vi "Globals_Settings_XLP80.vi"() -> ()   [LabVIEW 2021]
uses:
  XLP80_Datalog/XLP80_Datalog_TypeDefEnumLogselect.ctl
  <userlib>/PCAN Basic/Controls/Channel.ctl
  XLP80_General_Libs/Kirschenhofer_Libs/KH_DAQ 17.04/KH_DAQ_TypeDefs_Cluster AI.ctl
  XLP80_General_Libs/Kirschenhofer_Libs/KH_DAQ 17.04/KH_DAQ_TypeDefs_Messbereich.ctl
  XLP80_General_Libs/Kirschenhofer_Libs/KH EthernetIPConfig 17.14/KH EthernetIPConfig TypeDefs ModuleTyp.ctl
  XLP80_General_Libs/Kirschenhofer_Libs/KH_DAQ 17.04/KH_DAQ_TypeDefs_Bereich.ctl
  XLP80_General_Libs/Kirschenhofer_Libs/KH_DAQ 17.04/KH_DAQ_TypeDefs_Cluster AO.ctl
  XLP80_General_Libs/Kirschenhofer_Libs/KH_DAQ 17.04/Turck/KH_DAQ_TURCK_TypeDefs_Cluster DI.ctl
  XLP80_General_Libs/Kirschenhofer_Libs/KH_DAQ 17.04/Turck/KH_DAQ_TURCK_TypeDefs_Cluster DO.ctl
  <userlib>/PCAN Basic/PCANBasic.lvlib
panel:
  in  "Settings":T1(tab)=enum."Datalog"
  in  "EthernetIP ConfigFile":path=path "C:/Template/Results"
  in  "LogFile Path":path=path "C:/Template/Results"
  in  "Result Path":path=path "C:/Template/Results"
  in  "Settings Path":path=path "C:/Template/Settings"
  in  "MaxFileSize":i32
  in  "Logselect":T2[](array[typedef])
  in  "CVM Parameter":T3={"CVM Graph"={"CVM Warning"=0.0, "CVM Alarm"=0.0, "CVM GraphMin"=0.0, "CVM GraphMax"=0.0}, "Cells"=10, "StartChannel"="", "CVM Simulate"=TRUE, "CVMSimulation"={"CVMin"=0.0, "CVPeakNoise"=0.0}} {"CVMSimulation"."CVPeakNoise" min=0 max=1 scale=0.0..0.1; "CVMSimulation"."CVMin" min=0 max=1 scale=0.0..1.0}
  in  "ReadData":T4={"SheetName"="Header", "OffsetData"=2, "StartCell"="A3", "EndColumn"="D"}
  in  "ReadMetaData":T5={"SheetName"="Metadata", "NoOfRows"=6, "StartCell"="A1"}
  in  "Alarm Table Real":T6 {"Ena" format="%04b"; "Limits_III" format="%.2e"; "Limits II" format="%.2e"; "Limits I" format="%.2e"; "Index" max=63}
  in  "Alarm Table Bool":T7 {"Ena" format="%04b"; "Index" max=63}
  in  "EIP_AI":T8 {"Offset" format="%.4f"; "Phys Max" format="%.4f"; "Phys Min" format="%.4f"}
  in  "EIP_AO":T12 {"Offset" format="%.4f"; "Phys Max" format="%.4f"; "Phys Min" format="%.4f"}
  in  "EIP_DI":T13 {"Nr" max=63; "Chan" max=63}
  in  "EIP_DO":T14 {"Nr" max=63; "Chan" max=63}
  in  "CAN DBC":path
  in  "Peak Channel":T15=enum."PCAN_PCIBUS1"
  in  "Settings_CANWrite_Testmode_B":T16={"Signal Name"=["LV_en_p_cldn_amblimit_temp", "LV_en_p_cldn_amblimitoff_temp", "LV_en_p_cldn_cp_spd", "LV_en_p_cldn_rf_spd", "LV_en_p_cldn_rf_time", "LV_en_p_cldn_soclimit", "LV_en_p_cldn_time2off", "LV_en_p_cvm_diff_maxmin_lim", "LV_en_p_cvm_frequency", "LV_en_p_cvm_low_lim2", "LV_en_p_cvm_temperature", "LV_en_p_cvm_up_lim1", "LV_en_p_cvm_up_lim2", "LV_en_p_fcsd_etc_initrng_spd", "LV_en_p_fcsd_h2end_press", "LV_en_p_fcsd_hrbstp_spd", "LV_en_p_fcsu_bpv_opncls_time", "LV_en_p_fcsu_dcdc_currrampgrad", "LV_en_p_fcsu_dcdc_maxwrmup_curr", "LV_en_p_fcsu_dcdc_optime", "LV_en_p_fcsu_dcdc_preoptime", "LV_en_p_fcsu_etc_initspd", "LV_en_p_fcsu_ghu_strtpress1", "LV_en_p_fcsu_ghu_strtpress2", "LV_en_p_fcsu_h2_initpress", "LV_en_p_fcsu_h2_strtpress", "LV_en_p_fcsu_hrb_strtspd", "LV_en_p_fcsu_initmincellvolt", "LV_en_p_fcsu_mincellvolt_time", "LV_en_p_fcsu_pvrmp_incrclstime", "LV_en_p_fcsu_pvrmp_opntime", "LV_en_p_fcsu_pvrmp_strtclstime", "LV_en_p_fcsu_stk_deltamedlow_v", "LV_en_p_fcsu_stk_lowcellvolt", "LV_en_p_fcsu_stk_normopset_temp", "LV_en_p_hmi_bat_soc_limit_low", "LV_en_p_hmi_bat_soc_limit_ok", "LV_en_p_hmi_h2_leak_amb_ppm", "LV_en_p_hmi_h2_leak_exh_ppm", "LV_en_p_hmi_h2_leak_exh_s", "LV_en_p_hmi_h2tanklvl_displ", "LV_en_p_hmi_h2tanklvl_presslim", "LV_en_p_hmi_h2tanklvl_scale0", "LV_en_p_hmi_h2tanklvl_scale1", "LV_en_p_hrbo_a_valve_async_fact", "LV_en_p_hrbo_a_valve_i_fact", "LV_en_p_hrbo_a_valve_ot_fact", "LV_en_p_p_minucell_range1_time", "LV_en_p_p_minucell_range1_volt", "LV_en_p_p_minucell_range2_time", "LV_en_p_p_minucell_range2_volt", "LV_en_p_pc_uirangecell_time", "LV_en_p_pc_uirangecell_volt", "LV_en_p_power_out_fc_high", "LV_en_p_power_out_fc_low", "LV_en_p_rfc_hghvent_fanspd", "LV_en_p_rfc_nrmopbaseval_fanspd", "LV_en_p_rfc_srtstpvent_fanspd", "LV_en_p_soc_limit_fc_high", "LV_en_p_soc_limit_fc_low", "LV_en_p_soc_limit_fc_off", "LV_en_p_spdn_batlimit_curr", "LV_en_p_spdn_batlimit_time", "LV_en_p_tc_clpmpspd_idx0", "LV_en_p_tc_clpmpspd_idx1", "LV_en_p_tc_clpmpspd_idx2", "LV_en_P_TC_GHU_maxlowpress", "LV_en_P_TC_GHU_maxmidpress", "LV_en_P_TC_OTV_maxtankpress", "LV_en_p_wtlc_soc_lvl_perc", "LV_en_p_wtlc_soc_time2off_sec", "LV_P_CLDN_AMBlimit_Temp", "LV_P_CLDN_AMBlimitOff_Temp", "LV_P_CLDN_CP_Spd", "LV_P_CLDN_RF_Spd", "LV_P_CLDN_RF_Time", "LV_P_CLDN_SOClimit", "LV_P_CLDN_time2off", "LV_P_CVM_Diff_MaxMin_Lim", "LV_P_CVM_Frequency", "LV_P_CVM_Low_Lim2", "LV_P_CVM_Temperature", "LV_P_CVM_Up_Lim1", "LV_P_CVM_Up_Lim2", "LV_P_FCSD_ETC_InitRng_Spd", "LV_P_FCSD_H2end_Press", "LV_P_FCSD_HRBstp_Spd", "LV_P_FCSU_BPV_OpnCls_Time", "LV_P_FCSU_DCDC_CurrRampGrad", "LV_P_FCSU_DCDC_MaxWrmUp_Curr", "LV_P_FCSU_DCDC_OpTime", "LV_P_FCSU_DCDC_PreOpTime", "LV_P_FCSU_ETC_InitSpd", "LV_P_FCSU_GHU_StrtPress1", "LV_P_FCSU_GHU_StrtPress2", "LV_P_FCSU_H2_InitPress", "LV_P_FCSU_H2_Press_I_Ctrl", "LV_P_FCSU_H2_Press_P_Ctrl", "LV_P_FCSU_H2_StrtPress", "LV_P_FCSU_HRB_StrtSpd", "LV_P_FCSU_InitMinCellVolt", "LV_P_FCSU_MinCellVolt_Time", "LV_P_FCSU_PVrmp_IncrClsTime", "LV_P_FCSU_PVrmp_IniOpnTime", "LV_P_FCSU_PVrmp_StrtClsTime", "LV_P_FCSU_STK_DeltaMedLow_V", "LV_P_FCSU_STK_LowCellVolt", "LV_P_FCSU_STK_NormOpSet_Temp", "LV_P_HMI_BAT_SOC_Limit_low", "LV_P_HMI_BAT_SOC_Limit_ok", "LV_P_HMI_H2_leak_amb_ppm", "LV_P_HMI_H2_leak_exh_ppm", "LV_P_HMI_H2_leak_exh_s", "LV_P_HMI_H2TankLvl_Displ", "LV_P_HMI_H2TankLvl_PressLim", "LV_P_HMI_H2TankLvl_Scale0", "LV_P_HMI_H2TankLvl_Scale1", "LV_P_HRBo_a_Valve_Async_fact", "LV_P_HRBo_a_Valve_I_fact", "LV_P_HRBo_a_Valve_OT_fact", "LV_P_PC_MinUCell_range1_Time", "LV_P_PC_MinUCell_range1_Volt", "LV_P_PC_MinUCell_range2_Time", "LV_P_PC_MinUCell_range2_Volt", "LV_P_PC_UIrangeCell_Time", "LV_P_PC_UIrangeCell_Volt", "LV_P_Power_Out_FC_High", "LV_P_Power_Out_FC_Low", "LV_P_RFC_HghVent_FanSpd", "LV_P_RFC_NrmOpBaseVal_FanSpd", "LV_P_RFC_SrtStpVent_FanSpd", "LV_P_SOC_Limit_FC_High", "LV_P_SOC_Limit_FC_Low", "LV_P_SOC_Limit_FC_Off", "LV_P_SPDN_BATlimit_Curr", "LV_P_SPDN_BATlimit_Time", "LV_P_TC_ClPmpSpd_Amp0", "LV_P_TC_ClPmpSpd_Amp1", "LV_P_TC_ClPmpSpd_Amp2", "LV_P_TC_ClPmpSpd_perc0", "LV_P_TC_ClPmpSpd_perc1", "LV_P_TC_ClPmpSpd_perc2", "LV_P_TC_GHU_MaxLowPress", "LV_P_TC_GHU_MaxMidPress", "LV_P_TC_OTV_MaxTankPress", "LV_P_TC_StkIntT_I_Crtl_FanSpd", "LV_P_TC_StkIntT_P_Crtl_FanSpd", "LV_P_WTLC_SOC_Lvl", "LV_P_WTLC_SOC_time2off", "LV_Testmode_Select", "S80_BP_s_Taster_Start_Status", "S80_BP_s_Taster_Stop_Status"], "Description"=["", "", "", "", "", "", "", "", "", "", "", "", "", "", "", "", "", "", "", "", "", "", "", "", "", "", "", "", "", "", "", "", "", "", "", "", "", "", "", "", "", "", "", "", "", "", "", "", "", "", "", "", "", "", "", "", "", "", "", "", "", "", "", "", "", "", "", "", "", "", "", "", "", "", "", "", "", "", "", "", "", "", "", "", "", "", "", "", "", "", "", "", "", "", "", "", "", "", "", "", "", "", "", "", "", "", "", "", "", "", "", "", "", "", "", "", "", "", "", "", "", "", "", "", "", "", "", "", "", "", "", "", "", "", "", "", "", "", "", "", "", "", "", "", "", "", "", "", "", "", "", ""], "Unit"=["", "", "", "", "", "", "", "", "", "", "", "", "", "", "", "", "", "", "", "", "", "", "", "", "", "", "", "", "", "", "", "", "", "", "", "", "", "", "", "", "", "", "", "", "", "", "", "", "", "", "", "", "", "", "", "", "", "", "", "", "", "", "", "", "", "", "", "", "", "", "", "°C", "°C", "%", "%", "s", "%", "s", "V", "Hz", "V", "°C", "V", "V", "rpm", "kPa", "rpm", "s", "A/s", "A", "s", "s", "rpm", "kPa", "kPa", "kPa", "", "", "kPa", "rpm", "V", "s", "s", "s", "s", "V", "V", "°C", "%", "%", "ppm", "ppm", "s", "%", "kPa", "kPa", "kPa", "", "", "", "s", "V", "s", "V", "s", "V", "A", "A", "%", "%", "%", "%", "%", "%", "A", "s", "A", "A", "A", "%", "%", "%", "kPa", "kPa", "kPa", "", "", "%", "s", "", "", ""], "Default"=[0.0, 0.0, 0.0, 0.0, 0.0, 0.0, 0.0, 0.0, 0.0, 0.0, 0.0, 0.0, 0.0, 0.0, 0.0, 0.0, 0.0, 0.0, 0.0, 0.0, 0.0, 0.0, 0.0, 0.0, 0.0, 0.0, 0.0, 0.0, 0.0, 0.0, 0.0, 0.0, 0.0, 0.0, 0.0, 0.0, 0.0, 0.0, 0.0, 0.0, 0.0, 0.0, 0.0, 0.0, 0.0, 0.0, 0.0, 0.0, 0.0, 0.0, 0.0, 0.0, 0.0, 0.0, 0.0, 0.0, 0.0, 0.0, 0.0, 0.0, 0.0, 0.0, 0.0, 0.0, 0.0, 0.0, 0.0, 0.0, 0.0, 0.0, 0.0, 0.0, 0.0, 0.0, 0.0, 0.0, 0.0, 0.0, 0.0, 0.0, 0.0, 0.0, 0.0, 0.0, 0.0, 0.0, 0.0, 0.0, 0.0, 0.0, 0.0, 0.0, 0.0, 0.0, 0.0, 0.0, 0.0, 0.0, 0.0, 0.0, 0.0, 0.0, 0.0, 0.0, 0.0, 0.0, 0.0, 0.0, 0.0, 0.0, 0.0, 0.0, 0.0, 0.0, 0.0, 0.0, 0.0, 0.0, 0.0, 0.0, 0.0, 0.0, 0.0, 0.0, 0.0, 0.0, 0.0, 0.0, 0.0, 0.0, 0.0, 0.0, 0.0, 0.0, 0.0, 0.0, 0.0, 0.0, 0.0, 0.0, 0.0, 0.0, 0.0, 0.0, 0.0, 0.0, 0.0, 0.0, 0.0, 0.0, 0.0, 0.0], "Min"=[0.0, 0.0, 0.0, 0.0, 0.0, 0.0, 0.0, 0.0, 0.0, 0.0, 0.0, 0.0, 0.0, 0.0, 0.0, 0.0, 0.0, 0.0, 0.0, 0.0, 0.0, 0.0, 0.0, 0.0, 0.0, 0.0, 0.0, 0.0, 0.0, 0.0, 0.0, 0.0, 0.0, 0.0, 0.0, 0.0, 0.0, 0.0, 0.0, 0.0, 0.0, 0.0, 0.0, 0.0, 0.0, 0.0, 0.0, 0.0, 0.0, 0.0, 0.0, 0.0, 0.0, 0.0, 0.0, 0.0, 0.0, 0.0, 0.0, 0.0, 0.0, 0.0, 0.0, 0.0, 0.0, 0.0, 0.0, 0.0, 0.0, 0.0, 0.0, 0.0, 0.0, 0.0, 0.0, 0.0, 0.0, 0.0, 0.0, 0.0, 0.0, 0.0, 0.0, 0.0, 0.0, 0.0, 0.0, 0.0, 0.0, 0.0, 0.0, 0.0, 0.0, 0.0, 0.0, 0.0, 0.0, 0.0, 0.0, 0.0, 0.0, 0.0, 0.0, 0.0, 0.0, 0.0, 0.0, 0.0, 0.0, 0.0, 0.0, 0.0, 0.0, 0.0, 0.0, 0.0, 0.0, 0.0, 0.0, 0.0, 0.0, 0.0, 0.0, 0.0, 0.0, 0.0, 0.0, 0.0, 0.0, 0.0, 0.0, 0.0, 0.0, 0.0, 0.0, 0.0, 0.0, 0.0, 0.0, 0.0, 0.0, 0.0, 0.0, 0.0, 0.0, 0.0, 0.0, 0.0, 0.0, 0.0, 0.0, 0.0], "Max"=[100.0, 100.0, 100.0, 100.0, 100.0, 100.0, 100.0, 100.0, 100.0, 100.0, 100.0, 100.0, 100.0, 100.0, 100.0, 100.0, 100.0, 100.0, 100.0, 100.0, 100.0, 100.0, 100.0, 100.0, 100.0, 100.0, 100.0, 100.0, 100.0, 100.0, 100.0, 100.0, 100.0, 100.0, 100.0, 100.0, 100.0, 100.0, 100.0, 100.0, 100.0, 100.0, 100.0, 100.0, 100.0, 100.0, 100.0, 100.0, 100.0, 100.0, 100.0, 100.0, 100.0, 100.0, 100.0, 100.0, 100.0, 100.0, 100.0, 100.0, 100.0, 100.0, 100.0, 100.0, 100.0, 100.0, 100.0, 100.0, 100.0, 100.0, 100.0, 100.0, 100.0, 100.0, 100.0, 100.0, 100.0, 100.0, 100.0, 100.0, 100.0, 100.0, 100.0, 100.0, 100.0, 100.0, 100.0, 100.0, 100.0, 100.0, 100.0, 100.0, 100.0, 100.0, 100.0, 100.0, 100.0, 100.0, 100.0, 100.0, 100.0, 100.0, 100.0, 100.0, 100.0, 100.0, 100.0, 100.0, 100.0, 100.0, 100.0, 100.0, 100.0, 100.0, 100.0, 100.0, 100.0, 100.0, 100.0, 100.0, 100.0, 100.0, 100.0, 100.0, 100.0, 100.0, 100.0, 100.0, 100.0, 100.0, 100.0, 100.0, 100.0, 100.0, 100.0, 100.0, 100.0, 100.0, 100.0, 100.0, 100.0, 100.0, 100.0, 100.0, 100.0, 100.0, 100.0, 100.0, 100.0, 100.0, 100.0, 100.0], "Preconditions"=[FALSE, FALSE, FALSE, FALSE, FALSE, FALSE, FALSE, FALSE, FALSE, FALSE, FALSE, FALSE, FALSE, FALSE, FALSE, FALSE, FALSE, FALSE, FALSE, FALSE, FALSE, FALSE, FALSE, FALSE, FALSE], "HV & Software"=[FALSE, FALSE, FALSE, FALSE, FALSE, FALSE, FALSE, FALSE, FALSE, FALSE, FALSE, FALSE, FALSE, FALSE, FALSE, FALSE, FALSE, FALSE, FALSE, FALSE, FALSE, FALSE, FALSE, FALSE, FALSE], "Basis Funktion"=[FALSE, FALSE, FALSE, FALSE, FALSE, FALSE, FALSE, FALSE, FALSE, FALSE, FALSE, FALSE, FALSE, FALSE, FALSE, FALSE, FALSE, FALSE, FALSE, FALSE, FALSE, FALSE, FALSE, FALSE, FALSE], "Power Management"=[FALSE, FALSE, FALSE, FALSE, FALSE, FALSE, FALSE, FALSE, FALSE, FALSE, FALSE, FALSE, FALSE, FALSE, FALSE, FALSE, FALSE, FALSE, FALSE, FALSE, FALSE, FALSE, FALSE, FALSE, FALSE], "OperationMode"=[FALSE, FALSE, FALSE, FALSE, FALSE, FALSE, FALSE, FALSE, FALSE, FALSE, FALSE, FALSE, FALSE, FALSE, FALSE, FALSE, FALSE, FALSE, FALSE, FALSE, FALSE, FALSE, FALSE, FALSE, FALSE], "Shutdown"=[FALSE, FALSE, FALSE, FALSE, FALSE, FALSE, FALSE, FALSE, FALSE, FALSE, FALSE, FALSE, FALSE, FALSE, FALSE, FALSE, FALSE, FALSE, FALSE, FALSE, FALSE, FALSE, FALSE, FALSE, FALSE], "Alarm"=[FALSE, FALSE, FALSE, FALSE, FALSE, FALSE, FALSE, FALSE, FALSE, FALSE, FALSE, FALSE, FALSE, FALSE, FALSE, FALSE, FALSE, FALSE, FALSE, FALSE, FALSE, FALSE, FALSE, FALSE, FALSE], "LogEnable"=[FALSE, FALSE, FALSE, FALSE, FALSE, FALSE, FALSE, FALSE, FALSE, FALSE, FALSE, FALSE, FALSE, FALSE, FALSE, FALSE, FALSE, FALSE, FALSE, FALSE, FALSE, FALSE, FALSE, FALSE, FALSE]} {"Max" format="%.2f"; "Min" format="%.2f"; "Default" format="%.2f"}
  in  "Settings_CANRead_Testmode_B":T17 {"Max" format="%.2f"; "Min" format="%.2f"}
  in  "Settings_CANWrite_Testmode_A":T18={"Signal Name"=["LV_A_03_ETC_a_opCmd1_Error_Ack", "LV_A_03_ETC_a_opCmd1_Start_Stop", "LV_A_03_ETC_a_Speed_Set", "LV_A_11_HBV_a_Valve_Enable", "LV_A_11_HBV_a_Valve_Set", "LV_A_12_SIV_a_Valve_Enable", "LV_A_12_SIV_a_Valve_Set", "LV_A_13_SOV_a_Valve_Enable", "LV_A_13_SOV_a_Valve_Set", "LV_C_01_RF_a_FanSpeed", "LV_C_02_CP_a_RPM", "LV_E_74_ISO_a_Rq_D_IMC_STEST_SCR", "LV_E_75_HVP_a_Relais_Set", "LV_E_76_HVM_a_Relais_Set", "LV_H_31_OTV_a_Valve_Set", "LV_H_38_HSV_a_Valve_Set", "LV_H_42_HRB_a_FCCU_Spd_Rq", "LV_H_42_HRB_a_KNF_Speed_Rq", "LV_H_43_HDV_a_Dosing_Valve_Set", "LV_H_46_HRBo_a_Drain_Valve_Set", "LV_H_52_DV_a_Drain_Valve_Stack", "LV_H_53_PV_a_Purge_Valve_Stack", "LV_Testmode_Select", "S80_BP_s_Taster_Start_Status", "S80_BP_s_Taster_Stop_Status"], "Description"=["", "", "", "", "", "", "", "", "", "", "", "", "", "", "", "", "", "", "", "", "", "", "", "", ""], "Unit"=["", "", "rpm", "", "%", "", "%", "", "%", "%", "%", "", "", "", "", "", "rpm", "%", "%", "", "", "", "", "", ""], "Default"=[0.0, 0.0, 0.0, 0.0, 0.0, 0.0, 0.0, 0.0, 0.0, 0.0, 0.0, 0.0, 0.0, 0.0, 0.0, 0.0, 0.0, 0.0, 0.0, 0.0, 0.0, 0.0, 0.0, 0.0, 0.0], "Min"=[0.0, 0.0, 0.0, 0.0, 0.0, 0.0, 0.0, 0.0, 0.0, 0.0, 0.0, 0.0, 0.0, 0.0, 0.0, 0.0, 0.0, 0.0, 0.0, 0.0, 0.0, 0.0, 0.0, 0.0, 0.0], "Max"=[100.0, 100.0, 100.0, 100.0, 100.0, 100.0, 100.0, 100.0, 100.0, 100.0, 100.0, 100.0, 100.0, 100.0, 100.0, 100.0, 100.0, 100.0, 100.0, 100.0, 100.0, 100.0, 100.0, 100.0, 100.0], "TestmodeA"=[FALSE, FALSE, FALSE, FALSE, FALSE, FALSE, FALSE, FALSE, FALSE, FALSE, FALSE, FALSE, FALSE, FALSE, FALSE, FALSE, FALSE, FALSE, FALSE, FALSE, FALSE, FALSE, FALSE, FALSE, FALSE], "LogEnable"=[FALSE, FALSE, FALSE, FALSE, FALSE, FALSE, FALSE, FALSE, FALSE, FALSE, FALSE, FALSE, FALSE, FALSE, FALSE, FALSE, FALSE, FALSE, FALSE, FALSE, FALSE, FALSE, FALSE, FALSE, FALSE]} {"Max" format="%.2f"; "Min" format="%.2f"; "Default" format="%.2f"}
  in  "Settings_CANRead_Testmode_A":T19={"Signal Name"=["A03_ETC_a_CAN_Set_Baudrate", "A03_ETC_a_CAN_Set_Broadcast", "A03_ETC_a_CAN_Set_ID_Offset", "A03_ETC_a_CAN_Set_Termination", "A03_ETC_a_CAN_Set_Timeout", "A03_ETC_a_CAN_Set_Timeout_Dur", "A03_ETC_a_Diag_Rq_Select", "A03_ETC_a_Info_Rq_Select", "A03_ETC_a_opCmd1_Error_Ack", "A03_ETC_a_opCmd1_Start_Stop", "A03_ETC_a_opCmd2", "A03_ETC_a_Param_Rq_Select", "A03_ETC_a_Speed_Set", "A03_ETC_s_ArticleNumber", "A03_ETC_s_ArticleRevision", "A03_ETC_s_BootloaderVersion", "A03_ETC_s_Converter_Temperature", "A03_ETC_s_Diag_Select", "A03_ETC_s_Error_Code_1", "A03_ETC_s_Error_Code_2", "A03_ETC_s_FirmwareVersion", "A03_ETC_s_GasBearingCondition", "A03_ETC_s_HV_In_Voltage", "A03_ETC_s_Info_Select", "A03_ETC_s_Information_Code", "A03_ETC_s_LV_In_Voltage", "A03_ETC_s_Output_Power", "A03_ETC_s_Phase_Current", "A03_ETC_s_Phase_Current_Ref", "A03_ETC_s_Phase_Voltage", "A03_ETC_s_PT100_Temperature", "A03_ETC_s_Serial_Part_1", "A03_ETC_s_Serial_Part_2", "A03_ETC_s_Serial_Part_3", "A03_ETC_s_Speed_Actual", "A03_ETC_s_Speed_Reference", "A03_ETC_s_Status1", "A03_ETC_s_Status2", "A03_ETC_s_THC_Temperature", "A03_ETC_s_Warning_Code", "A11_HBV_a_Mode_Set", "A11_HBV_a_Valve_Set", "A11_HBV_s_Mode_Act", "A11_HBV_s_Valve_Act", "A12_SIV_a_Mode_Set", "A12_SIV_a_Valve_Set", "A12_SIV_s_Mode_Act", "A12_SIV_s_Valve_Act", "A13_SOV_a_Mode_Set", "A13_SOV_a_Valve_Set", "A13_SOV_s_Mode_Act", "A13_SOV_s_Valve_Act", "A14_HFM_s_AirMassFlow", "A14_HFM_s_Error_MassFlow", "A14_HFM_s_Error_Pressure", "A14_HFM_s_ErrorCode", "A14_HFM_s_Humidity", "A14_HFM_s_HumidTemperature", "A14_HFM_s_Pressure", "A14_HFM_s_Temperature", "A15_SI_s_Inlet_Pressure", "A16_SI_s_Inlet_Temperature", "A17_SO_s_Outlet_Pressure", "A17_SO_s_Outlet_Temperature", "A22_HSI_s_Humidity", "A23_HSO_s_Humidity", "A56_SO_s_Temperature", "C01_RF_a_FanSpeed", "C01_RF_s_Status", "C02_CP_a_RPM", "C04_DI_s_Temperature", "C06_ET_s_CoolLevelStatus", "C07_BAT_s_BatError_DataValid", "C07_BAT_s_BatError_Intern", "C07_BAT_s_BatError_Temperature", "C07_BAT_s_BatError_Voltage", "C07_BAT_s_Battery_Voltage", "C07_BAT_s_Board_Temperature", "C07_BAT_s_CECUError_Communicat", "C07_BAT_s_CECUError_Current", "C07_BAT_s_CECUError_Intern", "C07_BAT_s_CECUError_Reserved", "C07_BAT_s_CECUError_Service", "C07_BAT_s_CECUError_Supply", "C07_BAT_s_CECUError_Temperature", "C07_BAT_s_CECUError_Voltage", "C07_BAT_s_External_Chrg_Voltage", "C07_BAT_s_External_Load_Voltage", "C07_BAT_s_Max_Cell_Temperature", "C07_BAT_s_Max_Cell_Voltage", "C07_BAT_s_Min_Cell_Temperature", "C07_BAT_s_Min_Cell_Voltage", "C07_BAT_s_PreWarning_Current_H", "C07_BAT_s_PreWarning_SOC_Low", "C07_BAT_s_PreWarning_Temperature", "C07_BAT_s_PreWarning_Voltage_HL", "C07_BAT_s_State", "C07_BAT_s_System_Current", "C08_AMB_s_Humidity_Rel", "C08_AMB_s_Humidity_Spec", "C08_AMB_s_Pressure", "C08_AMB_s_Temperature", "C54_SI_s_Temperature", "C_07_BAT_s_SoC", "C_07_BAT_s_SoH", "E71_DC4880_a_Current_In_Set", "E71_DC4880_a_Current_Out_Set", "E71_DC4880_a_Mode_Control_On", "E71_DC4880_a_Mode_Precharge_On", "E71_DC4880_a_NMT_Function", "E71_DC4880_a_NMT_Node_ID", "E71_DC4880_a_Voltage_In_Set", "E71_DC4880_a_Voltage_Out_Set", "E71_DC4880_s_Current_In_Actual", "E71_DC4880_s_Current_Out_Actual", "E71_DC4880_s_NMT_State", "E71_DC4880_s_State_Control_OK", "E71_DC4880_s_State_Control_On", "E71_DC4880_s_State_Precharge_On", "E71_DC4880_s_Temperature_1_Act", "E71_DC4880_s_Temperature_2_Act", "E71_DC4880_s_Voltage_In_Actual", "E71_DC4880_s_Voltage_Out_Actual", "E72_DC8024_s_Voltage", "E73_DC8012_s_Voltage", "E74_ISO_a_CMD_Rq", "E74_ISO_a_Rq_D_IMC_MANUFACT_IDX", "E74_ISO_a_Rq_D_IMC_MEAN_FACTOR", "E74_ISO_a_Rq_D_IMC_R_ISOERR_THR", "E74_ISO_a_Rq_D_IMC_R_ISOWRN_THR", "E74_ISO_a_Rq_D_IMC_SELFTEST_SCR", "E74_ISO_a_Rq_D_IMC_VERSION_IDX", "E74_ISO_a_Rq_D_VIFC_HV_REL_CHG", "E74_ISO_a_Rq_D_VIFC_HV_RELAIS", "E74_ISO_a_Rq_D_VIFC_LOCK_MODE", "E74_ISO_a_Rq_D_VIFC_LOCK_PWD", "E74_ISO_a_Rq_D_VIFC_MEAS_MODE", "E74_ISO_a_Rq_D_VIFC_RELAIS_STAT", "E74_ISO_a_Rq_D_VIFC_VERSION_IDX", "E74_ISO_s_CMD_Resp", "E74_ISO_s_D_IMC_HV_1", "E74_ISO_s_D_IMC_HV_2", "E74_ISO_s_D_IMC_MANUFACT_DATA", "E74_ISO_s_D_IMC_MANUFACT_INDEX", "E74_ISO_s_D_IMC_MEAN_FACTOR", "E74_ISO_s_D_IMC_R_ISO", "E74_ISO_s_D_IMC_R_ISO_BIAS", "E74_ISO_s_D_IMC_R_ISO_CNT", "E74_ISO_s_D_IMC_R_ISO_ERR_THR1", "E74_ISO_s_D_IMC_R_ISO_ERR_THR2", "E74_ISO_s_D_IMC_R_ISO_WRN_THR1", "E74_ISO_s_D_IMC_R_ISO_WRN_THR2", "E74_ISO_s_D_IMC_SELFTEST_SCR", "E74_ISO_s_D_IMC_STATUS", "E74_ISO_s_D_IMC_STATUS_EXT", "E74_ISO_s_D_IMC_TEST_CNT", "E74_ISO_s_D_IMC_VERSION_Haupt", "E74_ISO_s_D_IMC_VERSION_INDEX", "E74_ISO_s_D_IMC_VERSION_Neben", "E74_ISO_s_D_IMD_ERROR_CODE", "E74_ISO_s_D_IMD_FAILED_CMD", "E74_ISO_s_D_VIFC_HV_RELAIS", "E74_ISO_s_D_VIFC_HV_RELAIS_ACT", "E74_ISO_s_D_VIFC_HV_RELAIS_CHG", "E74_ISO_s_D_VIFC_HV_RELAIS_STAT", "E74_ISO_s_D_VIFC_IMC_ALIVE", "E74_ISO_s_D_VIFC_LOCK_MODE", "E74_ISO_s_D_VIFC_MEASURE_MODE", "E74_ISO_s_D_VIFC_STATUS", "E74_ISO_s_D_VIFC_VERSION_Haupt", "E74_ISO_s_D_VIFC_VERSION_INDEX", "E74_ISO_s_D_VIFC_VERSION_Neben", "E74_ISO_s_IMC_R_ISO", "E74_ISO_s_IMC_STATUS_ErrChassis", "E74_ISO_s_IMC_STATUS_Isofehler", "E74_ISO_s_IMC_STATUS_Isowarnung", "E74_ISO_s_IMC_STATUS_Kalib", "E74_ISO_s_IMC_STATUS_Selbsttest", "E74_ISO_s_IMC_STATUS_Syststoer", "E74_ISO_s_Rq_D_IMC_MEAN_FACTOR", "E74_ISO_s_VIFC_STATUS_IMC_Alive", "E74_ISO_s_VIFC_STATUS_IMC_St_OA", "E74_ISO_s_VIFC_STATUS_IMC_St_PC", "E74_ISO_s_VIFC_STATUS_IsoAlt", "E74_ISO_s_VIFC_STATUS_Isomess", "E74_ISO_s_VIFC_STATUS_Stoer_IMC", "E74_ISO_s_VIFC_STATUS_VIFC_Cmd", "E75_HVP_a_Relais_Set", "E76_HVM_a_Relais_Set", "E95_DC2405_s_Voltage", "H31_OTV_a_Valve_Set", "H31_OTV_s_Pressure", "H31_OTV_s_Temperature", "H36_GHU_s_Pressure_1", "H37_GHU_s_Temperature_1", "H38_HSV_a_Valve_Set", "H40_GHU_s_Pressure_2", "H41_GHU_s_Temperature_2", "H42_HRB_a_FCCU_CRC", "H42_HRB_a_FCCU_Heating_Rq", "H42_HRB_a_FCCU_Spd_Rq", "H42_HRB_a_FCCU_SQC", "H42_HRB_s_ARB_Batt_Vltg_Err", "H42_HRB_s_ARB_Batt_Voltage", "H42_HRB_s_ARB_Blocked_Err", "H42_HRB_s_ARB_BrdgDrv_Err", "H42_HRB_s_ARB_E2E_Err", "H42_HRB_s_ARB_ECU_P_out", "H42_HRB_s_ARB_ECU_Temp", "H42_HRB_s_ARB_ECU_Temp_DrCnd", "H42_HRB_s_ARB_ECU_Temp_Err", "H42_HRB_s_ARB_ErrCRC", "H42_HRB_s_ARB_ErrSQC", "H42_HRB_s_ARB_I_D_Curr", "H42_HRB_s_ARB_I_Q_Curr", "H42_HRB_s_ARB_Init_Err", "H42_HRB_s_ARB_Mtr_Temp", "H42_HRB_s_ARB_Mtr_Temp_DrCnd", "H42_HRB_s_ARB_Mtr_Temp_Err", "H42_HRB_s_ARB_MtrNTCFlr_DrCnd", "H42_HRB_s_ARB_ShortToBat_Err", "H42_HRB_s_ARB_ShortToGround_Err", "H42_HRB_s_ARB_Spd", "H42_HRB_s_ARB_SpdDiff_DrCnd", "H42_HRB_s_ARB_SpdLimitRq_Err", "H42_HRB_s_ARB_SysState", "H42_HRB_s_ARB_Torque", "H42_HRB_s_ARB_U_D_Volt", "H42_HRB_s_ARB_U_Q_Volt", "H42_HRB_s_BrdgDrv_VCC_UV_Err", "H43_HDV_a_Dosing_Valve_Set", "H45_WT_s_WaterLevelStatus", "H46_HRBo_a_Drain_Valve_Set", "H51_STK_a_AmountOfModules_1002", "H51_STK_a_CAN_TerminatRes_1002", "H51_STK_a_CellsPerModule_1002", "H51_STK_a_CellVoltage_1001", "H51_STK_a_Command_1004", "H51_STK_a_CoreData_1001", "H51_STK_a_CoreData_Freq_1002", "H51_STK_a_DataLength_1001", "H51_STK_a_DataLength_1002", "H51_STK_a_DataLength_1003", "H51_STK_a_DataLength_1004", "H51_STK_a_DataLength_1006", "H51_STK_a_DataLength_100B", "H51_STK_a_DateTime_1002", "H51_STK_a_Diff_MaxMin_limit_1002", "H51_STK_a_FCCUResponse_1006", "H51_STK_a_Firmware_1001", "H51_STK_a_ID_1003", "H51_STK_a_ID_1004", "H51_STK_a_ID_H_1001", "H51_STK_a_ID_H_1002", "H51_STK_a_ID_H_100B", "H51_STK_a_ID_L_1001", "H51_STK_a_ID_L_1002", "H51_STK_a_ID_L_100B", "H51_STK_a_Logdata_1001", "H51_STK_a_Lower_Limit2_1002", "H51_STK_a_MasterNo_1002", "H51_STK_a_Modul_100B", "H51_STK_a_Monitoring_Flag_1003", "H51_STK_a_PosAtStack_1002", "H51_STK_a_StackSize_1002", "H51_STK_a_Temperature_1002", "H51_STK_a_Upper_Limit1_1002", "H51_STK_a_UpperLimit2_1002", "H51_STK_s_Amount_Slave_Modu_2000", "H51_STK_s_AmountofContactFailure", "H51_STK_s_AmountOfFrames_2002", "H51_STK_s_AmountOfFrames_2003", "H51_STK_s_AmountOfFrames_2005", "H51_STK_s_AmountOfFrames_2006", "H51_STK_s_AmountOfFrames_2011", "H51_STK_s_AverageTemp_2004", "H51_STK_s_CellContactNr10_2006", "H51_STK_s_CellContactNr11_2006", "H51_STK_s_CellContactNr12_2006", "H51_STK_s_CellContactNr13_2006", "H51_STK_s_CellContactNr14_2006", "H51_STK_s_CellContactNr15_2006", "H51_STK_s_CellContactNr16_2006", "H51_STK_s_CellContactNr17_2006", "H51_STK_s_CellContactNr18_2006", "H51_STK_s_CellContactNr19_2006", "H51_STK_s_CellContactNr1_2006", "H51_STK_s_CellContactNr20_2006", "H51_STK_s_CellContactNr21_2006", "H51_STK_s_CellContactNr22_2006", "H51_STK_s_CellContactNr23_2006", "H51_STK_s_CellContactNr24_2006", "H51_STK_s_CellContactNr25_2006", "H51_STK_s_CellContactNr26_2006", "H51_STK_s_CellContactNr27_2006", "H51_STK_s_CellContactNr28_2006", "H51_STK_s_CellContactNr29_2006", "H51_STK_s_CellContactNr2_2006", "H51_STK_s_CellContactNr30_2006", "H51_STK_s_CellContactNr31_2006", "H51_STK_s_CellContactNr32_2006", "H51_STK_s_CellContactNr33_2006", "H51_STK_s_CellContactNr34_2006", "H51_STK_s_CellContactNr35_2006", "H51_STK_s_CellContactNr36_2006", "H51_STK_s_CellContactNr37_2006", "H51_STK_s_CellContactNr38_2006", "H51_STK_s_CellContactNr39_2006", "H51_STK_s_CellContactNr3_2006", "H51_STK_s_CellContactNr40_2006", "H51_STK_s_CellContactNr41_2006", "H51_STK_s_CellContactNr42_2006", "H51_STK_s_CellContactNr43_2006", "H51_STK_s_CellContactNr44_2006", "H51_STK_s_CellContactNr45_2006", "H51_STK_s_CellContactNr46_2006", "H51_STK_s_CellContactNr47_2006", "H51_STK_s_CellContactNr48_2006", "H51_STK_s_CellContactNr49_2006", "H51_STK_s_CellContactNr4_2006", "H51_STK_s_CellContactNr50_2006", "H51_STK_s_CellContactNr51_2006", "H51_STK_s_CellContactNr52_2006", "H51_STK_s_CellContactNr53_2006", "H51_STK_s_CellContactNr54_2006", "H51_STK_s_CellContactNr55_2006", "H51_STK_s_CellContactNr56_2006", "H51_STK_s_CellContactNr57_2006", "H51_STK_s_CellContactNr58_2006", "H51_STK_s_CellContactNr59_2006", "H51_STK_s_CellContactNr5_2006", "H51_STK_s_CellContactNr60_2006", "H51_STK_s_CellContactNr61_2006", "H51_STK_s_CellContactNr62_2006", "H51_STK_s_CellContactNr63_2006", "H51_STK_s_CellContactNr64_2006", "H51_STK_s_CellContactNr65_2006", "H51_STK_s_CellContactNr66_2006", "H51_STK_s_CellContactNr67_2006", "H51_STK_s_CellContactNr68_2006", "H51_STK_s_CellContactNr69_2006", "H51_STK_s_CellContactNr6_2006", "H51_STK_s_CellContactNr70_2006", "H51_STK_s_CellContactNr71_2006", "H51_STK_s_CellContactNr7_2006", "H51_STK_s_CellContactNr8_2006", "H51_STK_s_CellContactNr9_2006", "H51_STK_s_CellNo_2ndlow_2003", "H51_STK_s_CellNo_highest_2003", "H51_STK_s_CellNo_lowest_2003", "H51_STK_s_CellVolt_001_2005", "H51_STK_s_CellVolt_002_2005", "H51_STK_s_CellVolt_003_2005", "H51_STK_s_CellVolt_004_2005", "H51_STK_s_CellVolt_005_2005", "H51_STK_s_CellVolt_006_2005", "H51_STK_s_CellVolt_007_2005", "H51_STK_s_CellVolt_008_2005", "H51_STK_s_CellVolt_009_2005", "H51_STK_s_CellVolt_010_2005", "H51_STK_s_CellVolt_011_2005", "H51_STK_s_CellVolt_012_2005", "H51_STK_s_CellVolt_013_2005", "H51_STK_s_CellVolt_014_2005", "H51_STK_s_CellVolt_015_2005", "H51_STK_s_CellVolt_016_2005", "H51_STK_s_CellVolt_017_2005", "H51_STK_s_CellVolt_018_2005", "H51_STK_s_CellVolt_019_2005", "H51_STK_s_CellVolt_020_2005", "H51_STK_s_CellVolt_021_2005", "H51_STK_s_CellVolt_022_2005", "H51_STK_s_CellVolt_023_2005", "H51_STK_s_CellVolt_024_2005", "H51_STK_s_CellVolt_025_2005", "H51_STK_s_CellVolt_026_2005", "H51_STK_s_CellVolt_027_2005", "H51_STK_s_CellVolt_028_2005", "H51_STK_s_CellVolt_029_2005", "H51_STK_s_CellVolt_030_2005", "H51_STK_s_CellVolt_031_2005", "H51_STK_s_CellVolt_032_2005", "H51_STK_s_CellVolt_033_2005", "H51_STK_s_CellVolt_034_2005", "H51_STK_s_CellVolt_035_2005", "H51_STK_s_CellVolt_036_2005", "H51_STK_s_CellVolt_037_2005", "H51_STK_s_CellVolt_038_2005", "H51_STK_s_CellVolt_039_2005", "H51_STK_s_CellVolt_040_2005", "H51_STK_s_CellVolt_041_2005", "H51_STK_s_CellVolt_042_2005", "H51_STK_s_CellVolt_043_2005", "H51_STK_s_CellVolt_044_2005", "H51_STK_s_CellVolt_045_2005", "H51_STK_s_CellVolt_046_2005", "H51_STK_s_CellVolt_047_2005", "H51_STK_s_CellVolt_048_2005", "H51_STK_s_CellVolt_049_2005", "H51_STK_s_CellVolt_050_2005", "H51_STK_s_CellVolt_051_2005", "H51_STK_s_CellVolt_052_2005", "H51_STK_s_CellVolt_053_2005", "H51_STK_s_CellVolt_054_2005", "H51_STK_s_CellVolt_055_2005", "H51_STK_s_CellVolt_056_2005", "H51_STK_s_CellVolt_057_2005", "H51_STK_s_CellVolt_058_2005", "H51_STK_s_CellVolt_059_2005", "H51_STK_s_CellVolt_060_2005", "H51_STK_s_CellVolt_061_2005", "H51_STK_s_CellVolt_062_2005", "H51_STK_s_CellVolt_063_2005", "H51_STK_s_CellVolt_064_2005", "H51_STK_s_CellVolt_065_2005", "H51_STK_s_CellVolt_066_2005", "H51_STK_s_CellVolt_067_2005", "H51_STK_s_CellVolt_068_2005", "H51_STK_s_CellVolt_069_2005", "H51_STK_s_CellVolt_070_2005", "H51_STK_s_CellVolt_071_2005", "H51_STK_s_CellVolt_2ndlow_2003", "H51_STK_s_CellVolt_follow_2ndlow", "H51_STK_s_CellVolt_follow_lowest", "H51_STK_s_CellVolt_highest_2003", "H51_STK_s_CellVolt_lowest_2003", "H51_STK_s_CellVolt_prev_2ndlow", "H51_STK_s_CellVolt_prev_lowest", "H51_STK_s_CellVoltage_ui16H_2004", "H51_STK_s_CellVoltage_ui16L_2004", "H51_STK_s_Contact_Cell_10_2010", "H51_STK_s_Contact_Cell_11_2010", "H51_STK_s_Contact_Cell_12_2010", "H51_STK_s_Contact_Cell_13_2010", "H51_STK_s_Contact_Cell_14_2010", "H51_STK_s_Contact_Cell_15_2010", "H51_STK_s_Contact_Cell_16_2010", "H51_STK_s_Contact_Cell_17_2010", "H51_STK_s_Contact_Cell_18_2010", "H51_STK_s_Contact_Cell_19_2010", "H51_STK_s_Contact_Cell_1_2010", "H51_STK_s_Contact_Cell_20_2010", "H51_STK_s_Contact_Cell_21_2010", "H51_STK_s_Contact_Cell_22_2010", "H51_STK_s_Contact_Cell_23_2010", "H51_STK_s_Contact_Cell_24_2010", "H51_STK_s_Contact_Cell_25_2010", "H51_STK_s_Contact_Cell_26_2010", "H51_STK_s_Contact_Cell_27_2010", "H51_STK_s_Contact_Cell_28_2010", "H51_STK_s_Contact_Cell_29_2010", "H51_STK_s_Contact_Cell_2_2010", "H51_STK_s_Contact_Cell_30_2010", "H51_STK_s_Contact_Cell_31_2010", "H51_STK_s_Contact_Cell_32_2010", "H51_STK_s_Contact_Cell_33_2010", "H51_STK_s_Contact_Cell_34_2010", "H51_STK_s_Contact_Cell_35_2010", "H51_STK_s_Contact_Cell_36_2010", "H51_STK_s_Contact_Cell_37_2010", "H51_STK_s_Contact_Cell_38_2010", "H51_STK_s_Contact_Cell_39_2010", "H51_STK_s_Contact_Cell_3_2010", "H51_STK_s_Contact_Cell_40_2010", "H51_STK_s_Contact_Cell_41_2010", "H51_STK_s_Contact_Cell_42_2010", "H51_STK_s_Contact_Cell_43_2010", "H51_STK_s_Contact_Cell_44_2010", "H51_STK_s_Contact_Cell_45_2010", "H51_STK_s_Contact_Cell_46_2010", "H51_STK_s_Contact_Cell_47_2010", "H51_STK_s_Contact_Cell_48_2010", "H51_STK_s_Contact_Cell_49_2010", "H51_STK_s_Contact_Cell_4_2010", "H51_STK_s_Contact_Cell_50_2010", "H51_STK_s_Contact_Cell_51_2010", "H51_STK_s_Contact_Cell_52_2010", "H51_STK_s_Contact_Cell_53_2010", "H51_STK_s_Contact_Cell_54_2010", "H51_STK_s_Contact_Cell_55_2010", "H51_STK_s_Contact_Cell_56_2010", "H51_STK_s_Contact_Cell_57_2010", "H51_STK_s_Contact_Cell_58_2010", "H51_STK_s_Contact_Cell_59_2010", "H51_STK_s_Contact_Cell_5_2010", "H51_STK_s_Contact_Cell_60_2010", "H51_STK_s_Contact_Cell_61_2010", "H51_STK_s_Contact_Cell_62_2010", "H51_STK_s_Contact_Cell_63_2010", "H51_STK_s_Contact_Cell_64_2010", "H51_STK_s_Contact_Cell_65_2010", "H51_STK_s_Contact_Cell_66_2010", "H51_STK_s_Contact_Cell_67_2010", "H51_STK_s_Contact_Cell_68_2010", "H51_STK_s_Contact_Cell_69_2010", "H51_STK_s_Contact_Cell_6_2010", "H51_STK_s_Contact_Cell_70_2010", "H51_STK_s_Contact_Cell_71_2010", "H51_STK_s_Contact_Cell_7_2010", "H51_STK_s_Contact_Cell_8_2010", "H51_STK_s_Contact_Cell_9_2010", "H51_STK_s_CVM_Firmw_Master_2002", "H51_STK_s_CVM_Firmw_Slave10_2002", "H51_STK_s_CVM_Firmw_Slave11_2002", "H51_STK_s_CVM_Firmw_Slave12_2002", "H51_STK_s_CVM_Firmw_Slave13_2002", "H51_STK_s_CVM_Firmw_Slave14_2002", "H51_STK_s_CVM_Firmw_Slave15_2002", "H51_STK_s_CVM_Firmw_Slave16_2002", "H51_STK_s_CVM_Firmw_Slave17_2002", "H51_STK_s_CVM_Firmw_Slave18_2002", "H51_STK_s_CVM_Firmw_Slave19_2002", "H51_STK_s_CVM_Firmw_Slave1_2002", "H51_STK_s_CVM_Firmw_Slave20_2002", "H51_STK_s_CVM_Firmw_Slave21_2002", "H51_STK_s_CVM_Firmw_Slave22_2002", "H51_STK_s_CVM_Firmw_Slave23_2002", "H51_STK_s_CVM_Firmw_Slave24_2002", "H51_STK_s_CVM_Firmw_Slave2_2002", "H51_STK_s_CVM_Firmw_Slave3_2002", "H51_STK_s_CVM_Firmw_Slave4_2002", "H51_STK_s_CVM_Firmw_Slave5_2002", "H51_STK_s_CVM_Firmw_Slave6_2002", "H51_STK_s_CVM_Firmw_Slave7_2002", "H51_STK_s_CVM_Firmw_Slave8_2002", "H51_STK_s_CVM_Firmw_Slave9_2002", "H51_STK_s_CVMResponse_200F", "H51_STK_s_DataLength_2000", "H51_STK_s_Datalength_2001", "H51_STK_s_Datalength_2004", "H51_STK_s_DataLength_200F", "H51_STK_s_DataLength_CVM_2010", "H51_STK_s_EventNo_2004", "H51_STK_s_FrameMux_2002", "H51_STK_s_FrameMux_2003", "H51_STK_s_FrameMux_2005", "H51_STK_s_FrameMux_2006", "H51_STK_s_FrameMux_2011", "H51_STK_s_FrameMux_CVM_2010", "H51_STK_s_ID_2001", "H51_STK_s_ID_H_2000", "H51_STK_s_ID_H_2002", "H51_STK_s_ID_H_200F", "H51_STK_s_ID_L_2000", "H51_STK_s_ID_L_2002", "H51_STK_s_ID_L_200F", "H51_STK_s_MasterBMS1REF1_2011", "H51_STK_s_MasterBMS1REF2_2011", "H51_STK_s_MasterBMS2REF1_2011", "H51_STK_s_MasterBMS2REF2_2011", "H51_STK_s_ModulHighestTemp_2003", "H51_STK_s_ModulNr_HighestTemp", "H51_STK_s_Mux_ID_2004", "H51_STK_s_RequestBit_2001", "H51_STK_s_Slave10BMS1REF1_2011", "H51_STK_s_Slave10BMS1REF2_2011", "H51_STK_s_Slave10BMS2REF1_2011", "H51_STK_s_Slave10BMS2REF2_2011", "H51_STK_s_Slave11BMS1REF1_2011", "H51_STK_s_Slave11BMS1REF2_2011", "H51_STK_s_Slave11BMS2REF1_2011", "H51_STK_s_Slave11BMS2REF2_2011", "H51_STK_s_Slave12BMS1REF1_2011", "H51_STK_s_Slave12BMS1REF2_2011", "H51_STK_s_Slave12BMS2REF1_2011", "H51_STK_s_Slave12BMS2REF2_2011", "H51_STK_s_Slave13BMS1REF1_2011", "H51_STK_s_Slave13BMS1REF2_2011", "H51_STK_s_Slave13BMS2REF1_2011", "H51_STK_s_Slave13BMS2REF2_2011", "H51_STK_s_Slave14BMS1REF1_2011", "H51_STK_s_Slave14BMS1REF2_2011", "H51_STK_s_Slave14BMS2REF1_2011", "H51_STK_s_Slave14BMS2REF2_2011", "H51_STK_s_Slave15BMS1REF1_2011", "H51_STK_s_Slave15BMS1REF2_2011", "H51_STK_s_Slave15BMS2REF1_2011", "H51_STK_s_Slave15BMS2REF2_2011", "H51_STK_s_Slave16BMS1REF1_2011", "H51_STK_s_Slave16BMS1REF2_2011", "H51_STK_s_Slave16BMS2REF1_2011", "H51_STK_s_Slave16BMS2REF2_2011", "H51_STK_s_Slave17BMS1REF1_2011", "H51_STK_s_Slave17BMS1REF2_2011", "H51_STK_s_Slave17BMS2REF1_2011", "H51_STK_s_Slave17BMS2REF2_2011", "H51_STK_s_Slave18BMS1REF1_2011", "H51_STK_s_Slave18BMS1REF2_2011", "H51_STK_s_Slave18BMS2REF1_2011", "H51_STK_s_Slave18BMS2REF2_2011", "H51_STK_s_Slave19BMS1REF1_2011", "H51_STK_s_Slave19BMS1REF2_2011", "H51_STK_s_Slave19BMS2REF1_2011", "H51_STK_s_Slave19BMS2REF2_2011", "H51_STK_s_Slave1BMS1REF1_2011", "H51_STK_s_Slave1BMS1REF2_2011", "H51_STK_s_Slave1BMS2REF1_2011", "H51_STK_s_Slave1BMS2REF2_2011", "H51_STK_s_Slave20BMS1REF1_2011", "H51_STK_s_Slave20BMS1REF2_2011", "H51_STK_s_Slave20BMS2REF1_2011", "H51_STK_s_Slave20BMS2REF2_2011", "H51_STK_s_Slave21BMS1REF1_2011", "H51_STK_s_Slave21BMS1REF2_2011", "H51_STK_s_Slave21BMS2REF1_2011", "H51_STK_s_Slave21BMS2REF2_2011", "H51_STK_s_Slave22BMS1REF1_2011", "H51_STK_s_Slave22BMS1REF2_2011", "H51_STK_s_Slave22BMS2REF1_2011", "H51_STK_s_Slave22BMS2REF2_2011", "H51_STK_s_Slave23BMS1REF1_2011", "H51_STK_s_Slave23BMS1REF2_2011", "H51_STK_s_Slave23BMS2REF1_2011", "H51_STK_s_Slave23BMS2REF2_2011", "H51_STK_s_Slave24BMS1REF1_2011", "H51_STK_s_Slave24BMS1REF2_2011", "H51_STK_s_Slave24BMS2REF1_2011", "H51_STK_s_Slave24BMS2REF2_2011", "H51_STK_s_Slave25BMS1REF1_2011", "H51_STK_s_Slave25BMS1REF2_2011", "H51_STK_s_Slave25BMS2REF1_2011", "H51_STK_s_Slave25BMS2REF2_2011", "H51_STK_s_Slave2BMS1REF1_2011", "H51_STK_s_Slave2BMS1REF2_2011", "H51_STK_s_Slave2BMS2REF1_2011", "H51_STK_s_Slave2BMS2REF2_2011", "H51_STK_s_Slave3BMS1REF1_2011", "H51_STK_s_Slave3BMS1REF2_2011", "H51_STK_s_Slave3BMS2REF1_2011", "H51_STK_s_Slave3BMS2REF2_2011", "H51_STK_s_Slave4BMS1REF1_2011", "H51_STK_s_Slave4BMS1REF2_2011", "H51_STK_s_Slave4BMS2REF1_2011", "H51_STK_s_Slave4BMS2REF2_2011", "H51_STK_s_Slave5BMS1REF1_2011", "H51_STK_s_Slave5BMS1REF2_2011", "H51_STK_s_Slave5BMS2REF1_2011", "H51_STK_s_Slave5BMS2REF2_2011", "H51_STK_s_Slave6BMS1REF1_2011", "H51_STK_s_Slave6BMS1REF2_2011", "H51_STK_s_Slave6BMS2REF1_2011", "H51_STK_s_Slave6BMS2REF2_2011", "H51_STK_s_Slave7BMS1REF1_2011", "H51_STK_s_Slave7BMS1REF2_2011", "H51_STK_s_Slave7BMS2REF1_2011", "H51_STK_s_Slave7BMS2REF2_2011", "H51_STK_s_Slave8BMS1REF1_2011", "H51_STK_s_Slave8BMS1REF2_2011", "H51_STK_s_Slave8BMS2REF1_2011", "H51_STK_s_Slave8BMS2REF2_2011", "H51_STK_s_Slave9BMS1REF1_2011", "H51_STK_s_Slave9BMS1REF2_2011", "H51_STK_s_Slave9BMS2REF1_2011", "H51_STK_s_Slave9BMS2REF2_2011", "H51_STK_s_Stat_CVM_Mastermo_2000", "H51_STK_s_TotalVoltage_2003", "H51_STK_s_Watchdog_2000", "H51_STK_s_ZellNo_2004", "H52_DV_a_Drain_Valve_Stack_Set", "H53_PV_a_Purge_Valve_Stack_Set", "H55_SI_s_Stack_Inlet_Pressure", "H62_HLD_s_1_CRC8", "H62_HLD_s_1_CycleCounter", "H62_HLD_s_1_Engineer_Info_1", "H62_HLD_s_1_Engineer_Info_2", "H62_HLD_s_1_Engineer_Info_3", "H62_HLD_s_1_Engineer_Info_4", "H62_HLD_s_1_H2_Concentration", "H62_HLD_s_1_HW_Type", "H62_HLD_s_1_HW_Version", "H62_HLD_s_1_Sensor_ErrorCode", "H62_HLD_s_1_SensorID", "H62_HLD_s_1_SW_Version_Main", "H62_HLD_s_1_SW_Version_Sub", "H62_HLD_s_2_CRC8", "H62_HLD_s_2_CycleCounter", "H62_HLD_s_2_Engineer_Info_1", "H62_HLD_s_2_Engineer_Info_2", "H62_HLD_s_2_Engineer_Info_3", "H62_HLD_s_2_Engineer_Info_4", "H62_HLD_s_2_H2_Concentration", "H62_HLD_s_2_HW_Type", "H62_HLD_s_2_HW_Version", "H62_HLD_s_2_Sensor_ErrorCode", "H62_HLD_s_2_SensorID", "H62_HLD_s_2_SW_Version_Main", "H62_HLD_s_2_SW_Version_Sub", "H63_HLD_s_1_CRC8", "H63_HLD_s_1_CycleCounter", "H63_HLD_s_1_Engineer_Info_1", "H63_HLD_s_1_Engineer_Info_2", "H63_HLD_s_1_Engineer_Info_3", "H63_HLD_s_1_Engineer_Info_4", "H63_HLD_s_1_H2_Concentration", "H63_HLD_s_1_HW_Type", "H63_HLD_s_1_HW_Version", "H63_HLD_s_1_Sensor_ErrorCode", "H63_HLD_s_1_SensorID", "H63_HLD_s_1_SW_Version_Main", "H63_HLD_s_1_SW_Version_Sub", "H63_HLD_s_2_CRC8", "H63_HLD_s_2_CycleCounter", "H63_HLD_s_2_Engineer_Info_1", "H63_HLD_s_2_Engineer_Info_2", "H63_HLD_s_2_Engineer_Info_3", "H63_HLD_s_2_Engineer_Info_4", "H63_HLD_s_2_H2_Concentration", "H63_HLD_s_2_HW_Type", "H63_HLD_s_2_HW_Version", "H63_HLD_s_2_Sensor_ErrorCode", "H63_HLD_s_2_SensorID", "H63_HLD_s_2_SW_Version_Main", "H63_HLD_s_2_SW_Version_Sub", "S80_BP_a_Bat_Control_LED_On", "S80_BP_a_Beep_On", "S80_BP_a_Distance_Horizontal", "S80_BP_a_Distance_Vertical", "S80_BP_a_FuelLevel_Display", "S80_BP_a_H2_Water_Ctrl_LED_On", "S80_BP_a_Leakage_LED_On", "S80_BP_a_Service_LED_On", "S80_BP_a_Taster_Start_LED_On", "S80_BP_a_Taster_Stop_LED_On", "S80_BP_a_WiFi_Status", "S80_BP_s_Taster_Start_Status", "S80_BP_s_Taster_Stop_Status", "S83_DCO_s_Wifi_Status", "S91_LV_Testmode"], "Description"=["", "", "", "", "", "", "", "", "", "", "", "", "", "", "", "", "", "", "", "", "", "", "", "", "", "", "", "", "", "", "", "", "", "", "", "", "", "", "", "", "", "", "", "", "", "", "", "", "", "", "", "", "", "", "", "", "", "", "", "", "", "", "", "", "", "", "", "", "", "", "", "", "", "", "", "", "", "", "", "", "", "", "", "", "", "", "", "", "", "", "", "", "", "", "", "", "", "", "", "", "", "", "", "", "", "", "", "", "", "", "", "", "", "", "", "", "", "", "", "", "", "", "", "", "", "", "", "", "", "", "", "", "", "", "", "", "", "", "", "", "", "", "", "", "", "", "", "", "", "", "", "", "", "", "", "", "", "", "", "", "", "", "", "", "", "", "", "", "", "", "", "", "", "", "", "", "", "", "", "", "", "", "", "", "", "", "", "", "", "", "", "", "", "", "", "", "", "", "", "", "", "", "", "", "", "", "", "", "", "", "", "", "", "", "", "", "", "", "", "", "", "", "", "", "", "", "", "", "", "", "", "", "", "", "", "", "", "", "", "", "", "", "", "", "", "", "", "", "", "", "", "", "", "", "", "", "", "", "", "", "", "", "", "", "", "", "", "", "", "", "", "", "", "", "", "", "", "", "", "", "", "", "", "", "", "", "", "", "", "", "", "", "", "", "", "", "", "", "", "", "", "", "", "", "", "", "", "", "", "", "", "", "", "", "", "", "", "", "", "", "", "", "", "", "", "", "", "", "", "", "", "", "", "", "", "", "", "", "", "", "", "", "", "", "", "", "", "", "", "", "", "", "", "", "", "", "", "", "", "", "", "", "", "", "", "", "", "", "", "", "", "", "", "", "", "", "", "", "", "", "", "", "", "", "", "", "", "", "", "", "", "", "", "", "", "", "", "", "", "", "", "", "", "", "", "", "", "", "", "", "", "", "", "", "", "", "", "", "", "", "", "", "", "", "", "", "", "", "", "", "", "", "", "", "", "", "", "", "", "", "", "", "", "", "", "", "", "", "", "", "", "", "", "", "", "", "", "", "", "", "", "", "", "", "", "", "", "", "", "", "", "", "", "", "", "", "", "", "", "", "", "", "", "", "", "", "", "", "", "", "", "", "", "", "", "", "", "", "", "", "", "", "", "", "", "", "", "", "", "", "", "", "", "", "", "", "", "", "", "", "", "", "", "", "", "", "", "", "", "", "", "", "", "", "", "", "", "", "", "", "", "", "", "", "", "", "", "", "", "", "", "", "", "", "", "", "", "", "", "", "", "", "", "", "", "", "", "", "", "", "", "", "", "", "", "", "", "", "", "", "", "", "", "", "", "", "", "", "", "", "", "", "", "", "", "", "", "", "", "", "", "", "", "", "", "", "", "", "", "", "", "", "", "", "", "", "", "", "", "", "", "", "", "", "", "", "", "", "", "", "", "", "", "", "", "", "", "", "", "", "", "", "", "", "", "", "", "", "", "", "", "", "", "", "", "", "", "", "", "", "", "", "", "", "", "", "", "", "", "", "", "", "", "", "", "", "", "", "", "", "", "", "", "", "", "", "", "", "", "", "", "", "", "", "", "", "", "", "", "", "", "", "", "", "", "", "", "", "", "", "", "", "", "", "", "", "", "", "", "", "", "", "", "", "", "", "", ""], "Unit"=["", "", "", "", "", "s", "", "", "", "", "", "", "rpm", "", "", "", "°C", "", "", "", "", "", "V", "", "", "V", "W", "A", "A", "V", "°C", "", "", "", "rpm", "rpm", "", "", "°C", "", "", "%", "", "%", "", "%", "", "%", "", "%", "", "%", "kg/h", "", "", "", "%RH", "°C", "kPa", "°C", "kPa", "°C", "kPa", "°C", "%RH", "%RH", "°C", "%", "", "%", "°C", "", "", "", "", "", "V", "°C", "", "", "", "", "", "", "", "", "V", "V", "°C", "V", "°C", "V", "", "", "", "", "", "A", "%RH", "g/kg", "kPa", "°C", "°C", "%", "%", "%", "%", "", "", "", "", "%", "%", "%", "%", "", "", "", "", "°C", "°C", "%", "%", "V", "V", "", "", "", "kOhm", "kOhm", "", "", "", "", "", "", "", "", "", "", "", "", "", "", "", "kOhm", "", "", "kOhm", "kOhm", "kOhm", "kOhm", "", "", "", "", "", "", "", "", "", "", "", "", "", "", "", "", "", "", "", "", "kOhm", "", "", "", "", "", "", "", "", "", "", "", "", "", "", "", "", "V", "", "kPa", "°C", "kPa", "°C", "", "kPa", "°C", "", "°C", "rpm", "", "", "V", "", "", "", "W", "°C", "", "", "", "", "A", "A", "", "°C", "", "", "", "", "", "rpm", "", "", "", "Nm", "V", "V", "", "%", "", "", "St.", "", "", "", "", "", "Hz", "", "", "", "", "", "", "", "", "", "", "", "", "", "", "", "", "", "", "", "mV", "", "", "", "Pos.", "Zellen", "", "mV", "mV", "St.", "", "", "", "", "", "", "°C", "", "", "", "", "", "", "", "", "", "", "", "", "", "", "", "", "", "", "", "", "", "", "", "", "", "", "", "", "", "", "", "", "", "", "", "", "", "", "", "", "", "", "", "", "", "", "", "", "", "", "", "", "", "", "", "", "", "", "", "", "", "", "", "", "", "", "", "", "", "", "", "Zelle", "Zelle", "Zelle", "mV", "mV", "mV", "mV", "mV", "mV", "mV", "mV", "mV", "mV", "mV", "mV", "mV", "mV", "mV", "mV", "mV", "mV", "mV", "mV", "mV", "mV", "mV", "mV", "mV", "mV", "mV", "mV", "mV", "mV", "mV", "mV", "mV", "mV", "mV", "mV", "mV", "mV", "mV", "mV", "mV", "mV", "mV", "mV", "mV", "mV", "mV", "mV", "mV", "mV", "mV", "mV", "mV", "mV", "mV", "mV", "mV", "mV", "mV", "mV", "mV", "mV", "mV", "mV", "mV", "mV", "mV", "mV", "mV", "mV", "mV", "mV", "mV", "mV", "mV", "mV", "mV", "mV", "mV", "mV", "", "", "", "", "", "", "", "", "", "", "", "", "", "", "", "", "", "", "", "", "", "", "", "", "", "", "", "", "", "", "", "", "", "", "", "", "", "", "", "", "", "", "", "", "", "", "", "", "", "", "", "", "", "", "", "", "", "", "", "", "", "", "", "", "", "", "", "", "", "", "", "", "", "", "", "", "", "", "", "", "", "", "", "", "", "", "", "", "", "", "", "", "", "", "", "", "", "", "", "", "", "", "", "", "", "", "", "", "", "", "", "", "", "", "", "", "", "", "", "", "", "", "", "", "", "", "", "", "", "", "", "", "", "", "", "", "", "", "", "", "", "", "", "", "", "", "", "", "", "", "", "", "", "", "", "", "", "", "", "", "", "", "", "", "", "", "", "", "", "", "", "", "", "", "", "", "", "", "", "", "", "", "", "", "", "", "", "", "", "", "", "", "", "", "", "", "", "", "", "", "", "", "", "", "", "", "", "", "", "", "", "", "", "", "", "", "", "", "", "", "", "", "", "", "", "mV", "", "", "", "", "kPa", "", "", "", "", "", "", "ppm", "", "", "", "", "", "", "", "", "", "", "", "", "ppm", "", "", "", "", "", "", "", "", "", "", "", "", "ppm", "", "", "", "", "", "", "", "", "", "", "", "", "ppm", "", "", "", "", "", "", "", "", "min", "min", "", "", "", "", "", "", "", "", "", "", ""], "Min"=[0.0, 0.0, 0.0, 0.0, 0.0, 0.0, 0.0, 0.0, 0.0, 0.0, 0.0, 0.0, 0.0, 0.0, 0.0, 0.0, 0.0, 0.0, 0.0, 0.0, 0.0, 0.0, 0.0, 0.0, 0.0], "Max"=[100.0, 100.0, 100.0, 100.0, 100.0, 100.0, 100.0, 100.0, 100.0, 100.0, 100.0, 100.0, 100.0, 100.0, 100.0, 100.0, 100.0, 100.0, 100.0, 100.0, 100.0, 100.0, 100.0, 100.0, 100.0], "TestmodeA"=[FALSE, FALSE, FALSE, FALSE, FALSE, FALSE, FALSE, FALSE, FALSE, FALSE, FALSE, FALSE, FALSE, FALSE, FALSE, FALSE, FALSE, FALSE, FALSE, FALSE, FALSE, FALSE, FALSE, FALSE, FALSE], "LogEnable"=[FALSE, FALSE, FALSE, FALSE, FALSE, FALSE, FALSE, FALSE, FALSE, FALSE, FALSE, FALSE, FALSE, FALSE, FALSE, FALSE, FALSE, FALSE, FALSE, FALSE, FALSE, FALSE, FALSE, FALSE, FALSE]} {"Max" format="%.2f"; "Min" format="%.2f"}
  in  "System":enum16{"GEN2_FM1", "GEN2_FM2"}(ring)
  in  "HWSimulation_EIP":bool=TRUE
  in  "HWSimulation_HH":bool=TRUE caption="Hardware Simulation EIP"
  in  "HWSimulation_EA_Stack":bool=TRUE caption="Hardware Simulation EIP"
  in  "HWSimulation_EA_Batterie":bool=TRUE caption="Hardware Simulation EIP"
  in  "HWSimulation_EA_Rekuperation":bool=TRUE caption="Hardware Simulation EIP"
  in  "ChartSettings 2":T20={"LineStyle"=[0, 0, 0, 0, 0, 0, 0, 0, 0, 0], "LineWidth"=[4, 4, 4, 6, 4, 4, 4, 4, 4, 4], "LineColor"=[4342338, 16711680, 34559, 7470974, 16759618, 5990723, 16776746, 46091, 8816262, 16711898], "SelectedPlot"=[0, 1, 2, 3, 4, 5, 6, 7, 8, 9], "Scales"=[1, 5, 3, 3, 3, 3, 3, 3, 3, 5], "Enabled"=[FALSE, FALSE, FALSE, FALSE, FALSE, FALSE, FALSE, FALSE, FALSE, FALSE]}
  in  "ChartSettings":T20={"LineStyle"=[0, 0, 0, 0, 0, 0, 0, 0, 0, 0], "LineWidth"=[4, 4, 4, 6, 4, 4, 4, 4, 4, 4], "LineColor"=[4342338, 16711680, 34559, 7470974, 16759618, 5990723, 16776746, 46091, 8816262, 16711898], "SelectedPlot"=[0, 1, 2, 3, 4, 5, 6, 7, 8, 9], "Scales"=[1, 5, 3, 3, 3, 3, 3, 3, 3, 5], "Enabled"=[FALSE, FALSE, FALSE, FALSE, FALSE, FALSE, FALSE, FALSE, FALSE, FALSE]}
  in  "Developer Mode":bool=TRUE caption="Developper Mode"
  in  "Logfile":bool
  in  "HWSimulation_CAN":bool=TRUE caption="Hardware Simulation EIP"
  # "Paths"
  # "1\n2\n3\n4\n5\n6\n7\n8\n9\n10\n11\n12\n13\n14\n15\n16\n17\n18\n19\n20\n21\n22\n23\n24\n25"
  # "bytes"
  # "WaitingToStart\nNormalOperation\nShutdown\nNotAus"
  # "WaitingToStart\nNormalOperation\nShutdown\nNotAus"
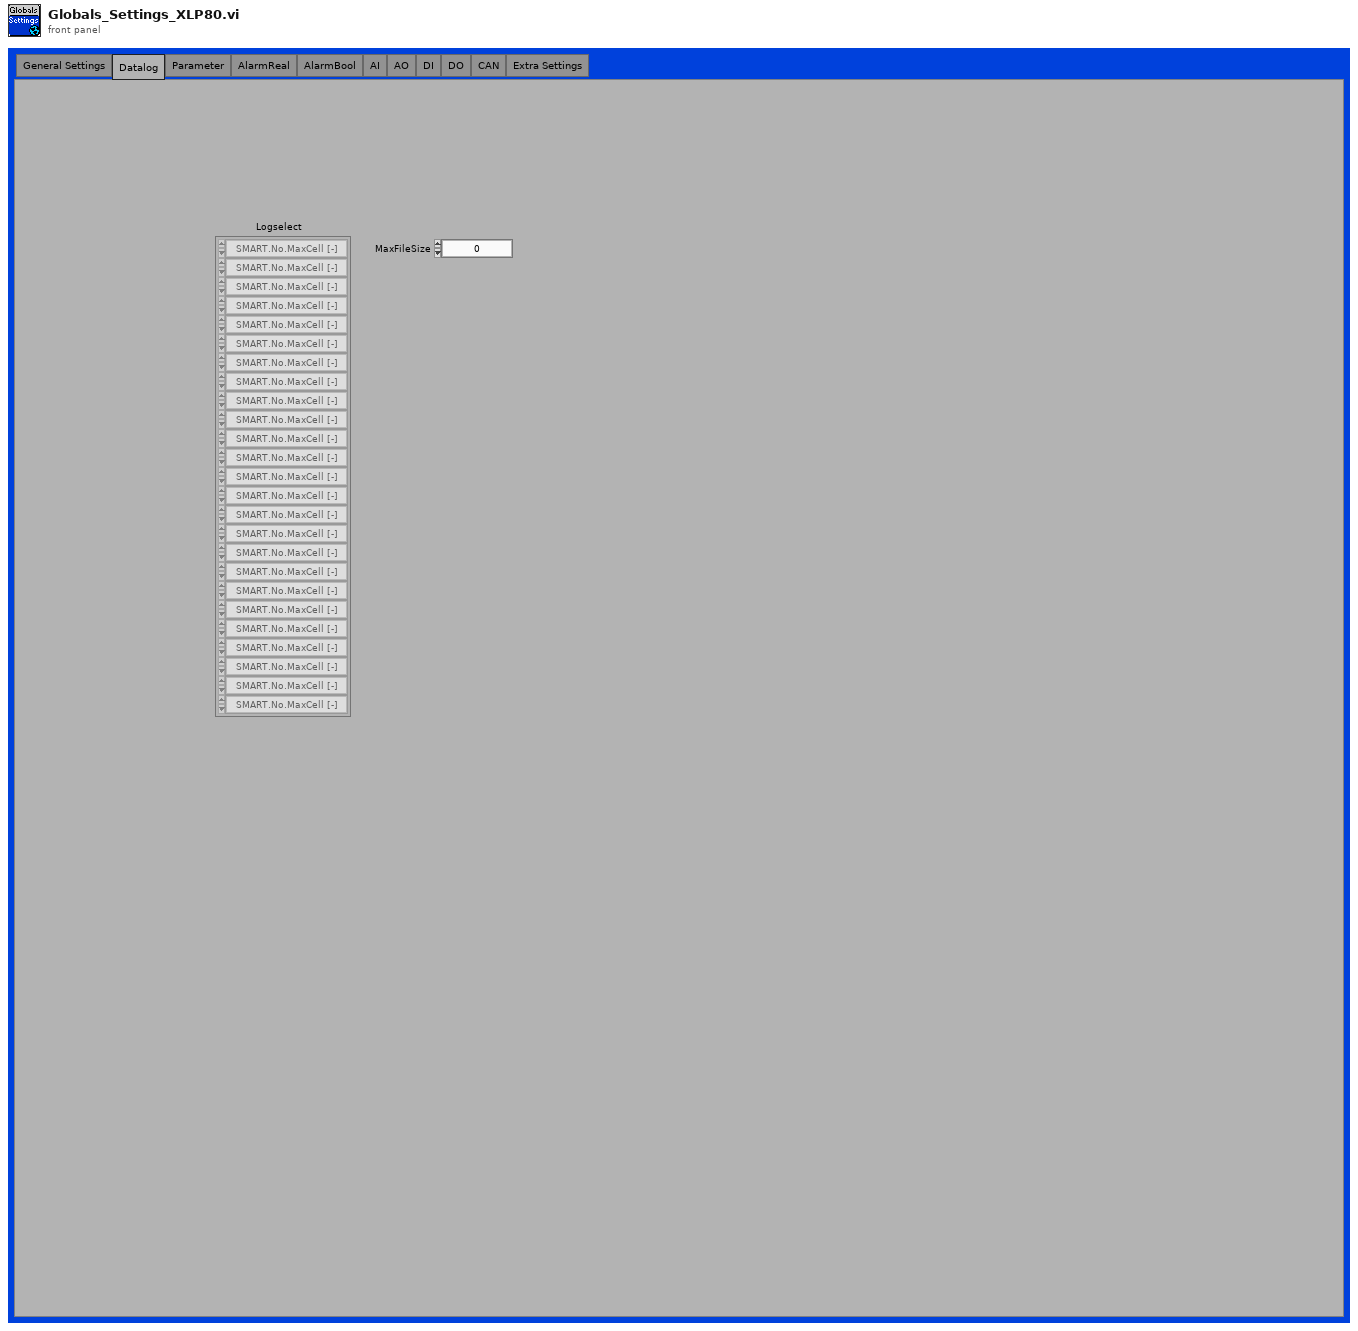
[diagram p1: front panel]
types:
  T1 = enum32{"General Settings", "Datalog", "Parameter", "AlarmReal", "AlarmBool", "AI", "AO", "DI", "DO", "CAN", "Extra Settings"}
  T2 = typedef "XLP80_Datalog_TypeDefEnumLogselect.ctl" = enum16{"SMART.No.MaxCell [-]", "SMART.No.MinCell [-]", "SMART.U.S.AveCell [V]", "SMART.U.S.CVM [V]", "SMART.U.S.MaxCell [V]", "SMART.U.S.MinCell [V]"}
  T3 = cluster{"CVM Graph":cluster{"CVM Warning":sgl, "CVM Alarm":sgl, "CVM GraphMin":sgl, "CVM GraphMax":sgl}, "Cells":i32, "StartChannel":string, "CVM Simulate":bool, "CVMSimulation":cluster{"CVMin":sgl, "CVPeakNoise":sgl}}
  T4 = cluster{"SheetName":string, "OffsetData":i32, "StartCell":string, "EndColumn":string}
  T5 = cluster{"SheetName":string, "NoOfRows":i32, "StartCell":string}
  T6 = cluster{"Name":string[], "Index":i32[], "Ena":u32[], "Limits I":sgl[][], "Delays_I":i32[][], "Limits II":sgl[][], "Delays_II":i32[][], "Limits_III":sgl[][], "Delays_III":i32[][], "Message":string[]}
  T7 = cluster{"Name":string[], "Index":i32[], "Ena":u32[], "Alarm_Cond":bool[], "I":bool[], "Delay_I":i32[], "II":bool[], "Delay_II":i32[], "III":bool[], "Delay_III":i32[], "Message":string[]}
  T8 = typedef "KH_DAQ_TypeDefs_Cluster AI.ctl" = cluster{"Signal Name":string[], "Description":string[], "Phys Unit":string[], "Messbereich":T9[], "Chan":u16[], "Phys Min":sgl[], "Phys Max":sgl[], "Offset":sgl[], "Nr":u16[], "SensorType 2":T10[], "Bereich":T11[]}
  T9 = typedef "KH_DAQ_TypeDefs_Messbereich.ctl" = enum16{"-10V ... +10V", "0V ... +10V", "+2V ... +10V", "0V ... +5V", "+1V ... +5V", "-1V ... +1V", "-500mV ... +500mV", "-100mV ... +100mV", "-50mV ... +50mV", "0mA ... +20mA", "+4mA ... +20mA", "-20mA ... +20mA", "0 Ohm ... 100 Ohm", "0 Ohm ... 400 Ohm", "0 Ohm ... 2000 Ohm", "0 Ohm ... 4000 Ohm", "-200°C ... 150°C PT100", "-200°C ... 150°C PT200", "-200°C ... 150°C PT500", "-200°C ... 150°C PT1000", "-60°C ... 150°C Ni100", "-60°C ... 150°C Ni1000", "-200°C ... 850°C PT100", "-200°C ... 850°C PT200", "-200°C ... 850°C PT500", "-200°C ... 850°C PT1000", "-50°C ... 250°C Ni100", "-50°C ... 250° Ni 1000"}
  T10 = typedef "KH EthernetIPConfig TypeDefs ModuleTyp.ctl" = enum16{"TBEN-S2-4AI", "TBEN-S1-8DXP", "TBEN-S2-2RFID-4DXP", "TBEN-S2-4AO", "TBEN-S2-4IOL"}
  T11 = typedef "KH_DAQ_TypeDefs_Bereich.ctl" = enum16{"Standard", "extended Range", "NE43", ""}
  T12 = typedef "KH_DAQ_TypeDefs_Cluster AO.ctl" = cluster{"Signal Name":string[], "Description":string[], "Phys Unit":string[], "Messbereich":T9[], "Chan":u16[], "Phys Min":sgl[], "Phys Max":sgl[], "Offset":sgl[], "Nr":u16[], "SensorType 2":T10[], "Bereich":T11[], "Default":sgl[]}
  T13 = typedef "KH_DAQ_TURCK_TypeDefs_Cluster DI.ctl" = cluster{"Signal Name":string[], "Description":string[], "Chan":u16[], "Inv":bool[], "Nr":u16[], "SensorType":T10[]}
  T14 = typedef "KH_DAQ_TURCK_TypeDefs_Cluster DO.ctl" = cluster{"Def":bool[], "Signal Name":string[], "Description":string[], "Chan":u16[], "Inv":bool[], "Nr":u16[], "SensorType":T10[]}
  T15 = typedef "PCANBasic.lvlib/Channel.ctl" = enum16{"PCAN_NONEBUS", "not used1", "not used2", "not used3", "not used4", "not used5", "not used6", "not used7", "not used8", "not used9", "not used10", "not used11", "not used12", "not used13", "not used14", "not used15", "not used16", "not used17", "not used18", "not used19", "not used20", "not used21", "not used22", "not used23", "not used24", "not used25", "not used26", "not used27", "not used28", "not used29", "not used30", "not used31", "not used32", "PCAN_ISABUS1", "PCAN_ISABUS2", "PCAN_ISABUS3", "PCAN_ISABUS4", "PCAN_ISABUS5", "PCAN_ISABUS6", "PCAN_ISABUS7", "PCAN_ISABUS8", "not used41", "not used42", "not used43", "not used44", "not used45", "not used46", "not used47", "not used48", "PCAN_DNGBUS1", "not used50", "not used51", "not used52", "not used53", "not used54", "not used55", "not used56", "not used57", "not used58", "not used59", "not used60", "not used61", "not used62", "not used63", "not used64", "PCAN_PCIBUS1", "PCAN_PCIBUS2", "PCAN_PCIBUS3", "PCAN_PCIBUS4", "PCAN_PCIBUS5", "PCAN_PCIBUS6", "PCAN_PCIBUS7", "PCAN_PCIBUS8", "not used73", "not used74", "not used75", "not used76", "not used77", "not used78", "not used79", "not used80", "PCAN_USBBUS1", "PCAN_USBBUS2", "PCAN_USBBUS3", "PCAN_USBBUS4", "PCAN_USBBUS5", "PCAN_USBBUS6", "PCAN_USBBUS7", "PCAN_USBBUS8", "Not used89", "Not used90", "Not used91", "Not used92", "Not used93", "Not used94", "Not used95", "Not used96", "PCAN_PCCBUS1", "PCAN_PCCBUS2"}
  T16 = cluster{"Signal Name":string[], "Description":string[], "Unit":string[], "Default":dbl[], "Min":dbl[], "Max":dbl[], "Preconditions":bool[], "HV & Software":bool[], "Basis Funktion":bool[], "Power Management":bool[], "OperationMode":bool[], "Shutdown":bool[], "Alarm":bool[], "LogEnable":bool[]}
  T17 = cluster{"Signal Name":string[], "Description":string[], "Unit":string[], "Min":dbl[], "Max":dbl[], "HV & Software":bool[], "Basis Funktion":bool[], "Power Management":bool[], "OperationMode":bool[], "Shutdown":bool[], "Alarm":bool[], "LogEnable":bool[]}
  T18 = cluster{"Signal Name":string[], "Description":string[], "Unit":string[], "Default":dbl[], "Min":dbl[], "Max":dbl[], "TestmodeA":bool[], "LogEnable":bool[]}
  T19 = cluster{"Signal Name":string[], "Description":string[], "Unit":string[], "Min":dbl[], "Max":dbl[], "TestmodeA":bool[], "LogEnable":bool[]}
  T20 = cluster{"LineStyle":u8[], "LineWidth":u8[], "LineColor":u32[], "SelectedPlot":i32[], "Scales":u16[], "Enabled":bool[]}
diagram:
